vi "cancel_goal_bool_msg.vi"(8 "error in (no error)":errorcluster caption="错误输入（无错误）", 10 "值(信号)":bool, 11 "RemoteP3AT输入":refnum<class "RemoteP3AT.lvclass">) -> (0 "error out":errorcluster caption="错误输出", 3 "RemoteP3AT输出":refnum<class "RemoteP3AT.lvclass">)   [LabVIEW 2014, in "RemoteP3AT.lvlib" / "RemoteP3AT.lvclass"]
uses:
  RemoteP3AT.lvclass
  RemoteP3AT.lvclass/RemoteP3AT.ctl
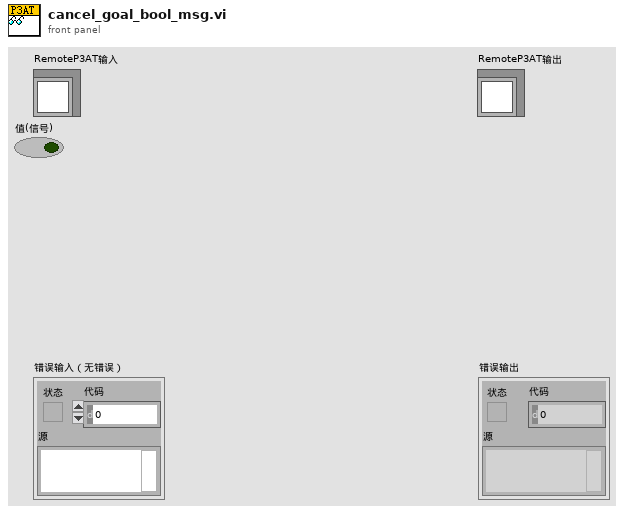
[diagram p1: front panel]
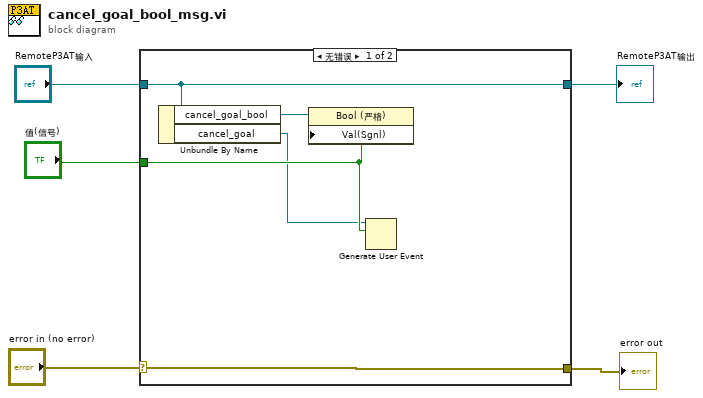
[diagram p0: block diagram]
diagram:
  n1 = case shown="无错误" "error in (no error)" {
    selector: "error in (no error)" -> [w10 w11]
    tunnel: [w10 w11] -> w4
    tunnel: [w9 w12] -> w2
    tunnel: "RemoteP3AT输入" -> [w9 w12]
    tunnel: "值(信号)" -> [w7 _]
    frame No Error {
      n2 = Unbundle By Name(w9) -> ("cancel_goal_bool"=w8:refnum<vi>, "cancel_goal"=w6:refnum<user-event>)
      n3 = property class="Bool (严格)"(reference=w8, "Val(Sgnl)"=w7) -> ()  [unwired: 1 in, 2 out]
      n4 = Generate User Event(user event=w6, event data cluster=w7) -> ()  [unwired: 2 in, 2 out]
    }
    frame Error {
    }
  }
  "error out" <- w4
  "RemoteP3AT输出" <- w2
